vi "Filter vi.lib VIs.vi"(8 "Error In":errorcluster, 11 "VIs In":T1[](array[typedef])) -> (0 "Error Out":errorcluster, 3 "VIs Out":T1[](array[typedef]))   [LabVIEW 2017, in "Bookmark Manager.lvlib"]
uses:
  Bookmark Manager.lvlib
  VI Information.ctl
  Application Information.ctl
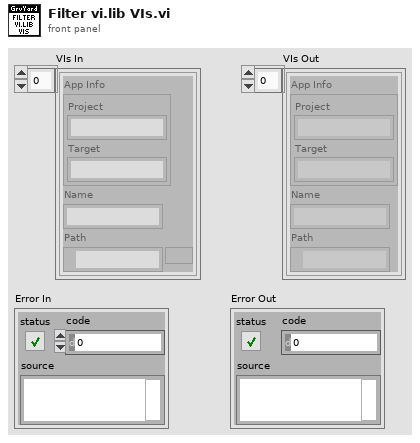
[diagram p1: front panel]
types:
  T1 = typedef "Bookmark Manager.lvlib/VI Information.ctl" = cluster{"App Info":T2, "Name":string, "Path":path}
  T2 = typedef "Bookmark Manager.lvlib/Application Information.ctl" = cluster{"Project":string, "Target":string}
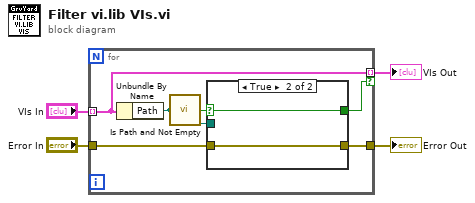
[diagram p0: block diagram]
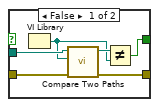
[diagram p2: hidden frame]
diagram:
  n1 = for {
    tunnel: "VIs In" -> [w6] mode=indexing
    tunnel: "Error In" -> [w8]
    tunnel: [w7] -> w4
    tunnel: [w6] -> w1 mode=indexing if=w5
    n2 = Unbundle By Name(w6) -> ("Path"=w9:path)
    n3 = call <vilib>:"Is Path and Not Empty.vi"("path"=w9) -> ("Is Path and Not Empty?"=w10:bool)  [unwired: 4 in]
    n4 = case shown="True" w10 {
      selector: w10 -> [_ w17]
      tunnel: w9 -> [w16 _]
      tunnel: w8 -> [w15 w18]
      tunnel: [w14 w18] -> w7
      tunnel: [w11 w17] -> w5
      frame False {
        n5 = VI Library() -> (path=w12:path)
        n6 = call <vilib>:"Compare Two Paths.vi"("error in (no error)"=w15, "Path 2"=w12, "Path 1"=w16) -> ("error out"=w14:errorcluster, "Relative Path from 1 to 2"=w13:path)  [unwired: 5 in, 2 out]
        n7 = Not Equal?(x=w13, y=w12) -> (x != y?=w11:bool)
      }
      frame True {
      }
    }
  }
  "Error Out" <- w4
  "VIs Out" <- w1
